vi "Verify Fiducial Positions.vi"(6 "Procedure Type":T1(ring)=enum."Gluing Verify Fiducials", 8 "error in":errorcluster, 9 "Path Fiducials":T8(array[cluster]), 10 "Module Fiducials":T6(array[cluster])) -> (0 "error out":errorcluster, 2 "All Good":bool)   [LabVIEW 2011]
uses:
  Shared Components/Utils/Type Definitions/Part Fiducials.ctl
  Shared Components/Utils/Type Definitions/Fiducial Image.ctl
  Shared Components/Vec3d Class/Vec3d Class.lvclass
  Shared Components/Utils/Type Definitions/Physical Image.ctl
  <vilib>/vision/Image Controls.llb/IMAQ Image.ctl
  Shared Components/Utils/Type Definitions/Fiducial with Source.ctl
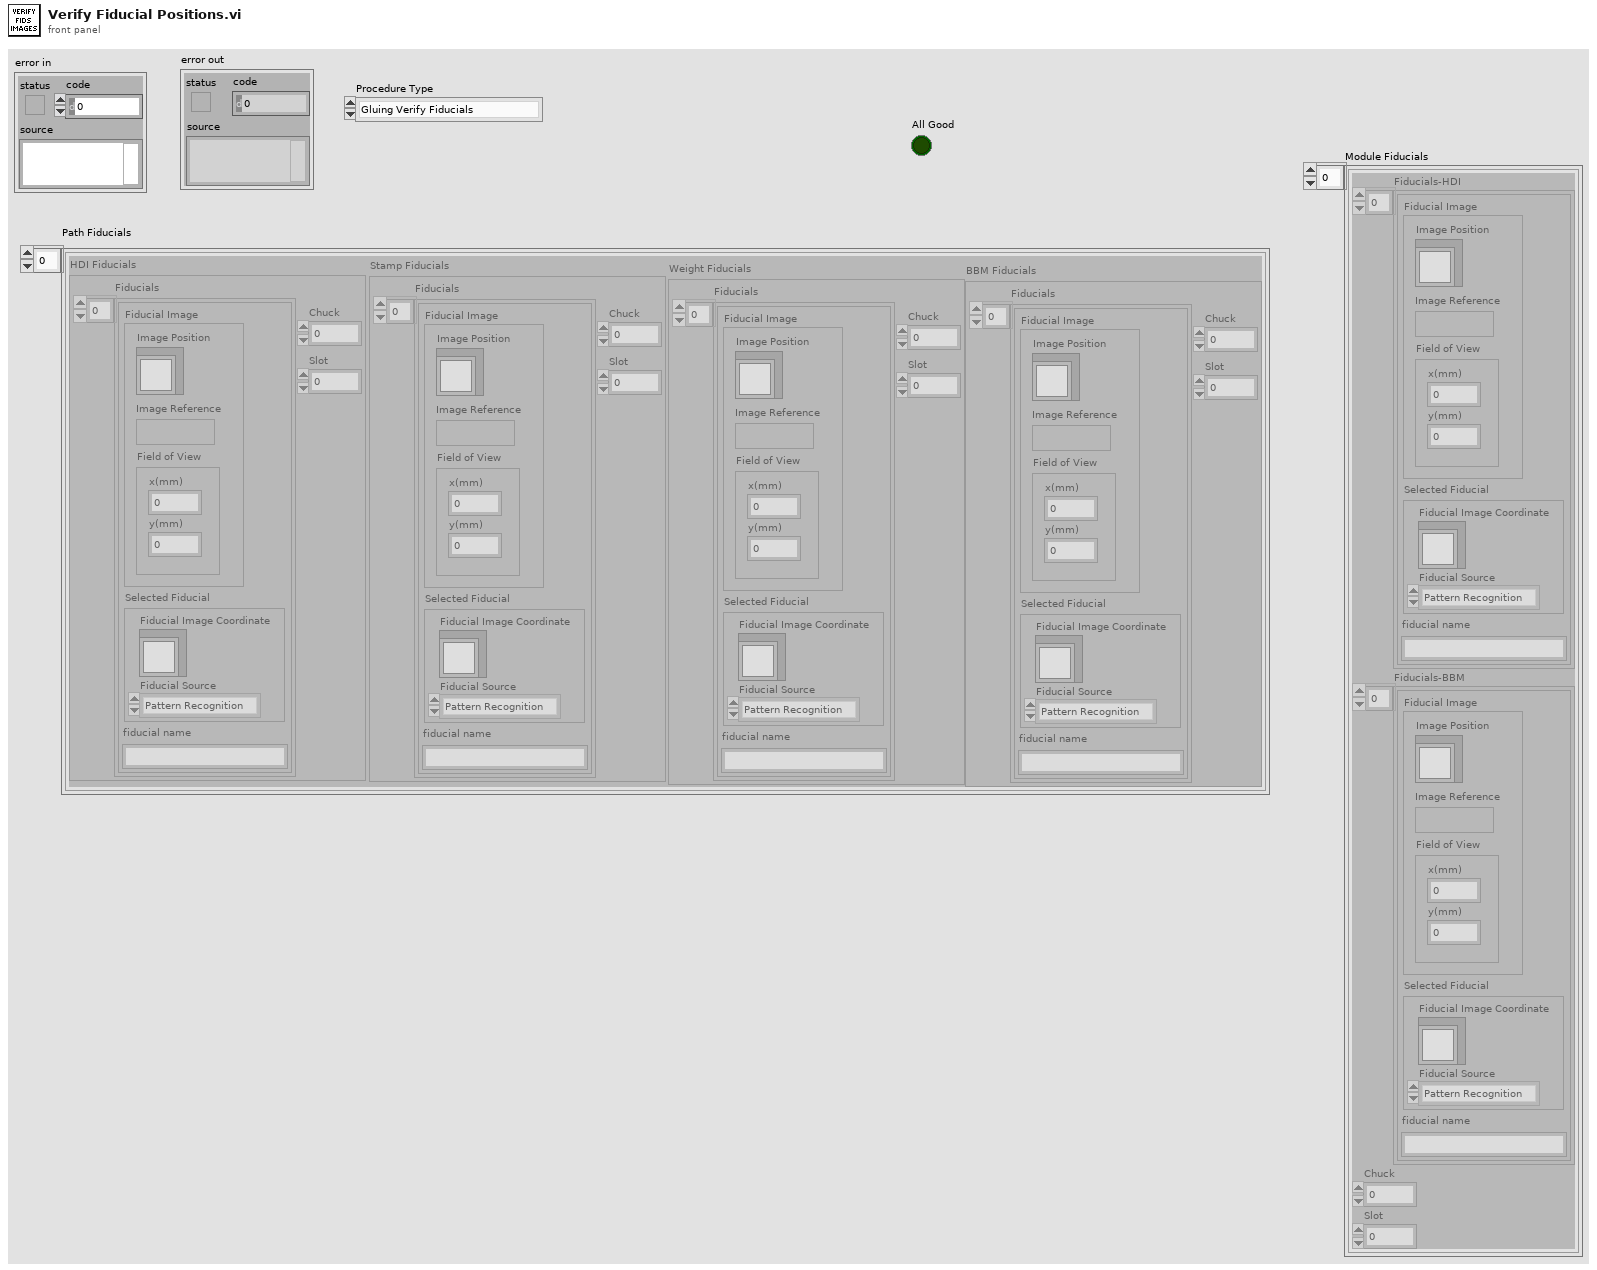
[diagram p1: front panel]
types:
  T1 = enum16{"Potting Verify Fiducials", "Gluing Verify Fiducials"}
  T2 = typedef "Fiducial Image.ctl" = cluster{"Fiducial Image":T3, "Selected Fiducial":T5, "fiducial name":string}
  T3 = typedef "Physical Image.ctl" = cluster{"Image Position":refnum<class "Vec3d Class.lvclass">, "Image Reference":T4, "Field of View":cluster{"x(mm)":dbl, "y(mm)":dbl}}
  T4 = typedef "IMAQ Image.ctl" = refnum<image>
  T5 = typedef "Fiducial with Source.ctl" = cluster{"Fiducial Image Coordinate":refnum<class "Vec3d Class.lvclass">, "Fiducial Source":enum16{"Pattern Recognition", "User", "Error", "Default"}}
  T6 = cluster{"Fiducials-HDI":T2[], "Fiducials-BBM":T2[], "Chuck":i32, "Slot":i32}[]
  T7 = typedef "Part Fiducials.ctl" = cluster{"Fiducials":T2[], "Chuck":i32, "Slot":i32}
  T8 = cluster{"HDI Fiducials":T7, "Stamp Fiducials":T7, "Weight Fiducials":T7, "BBM Fiducials":T7}[]
  T9 = enum16{"Pattern Recognition", "User", "Error", "Default"}
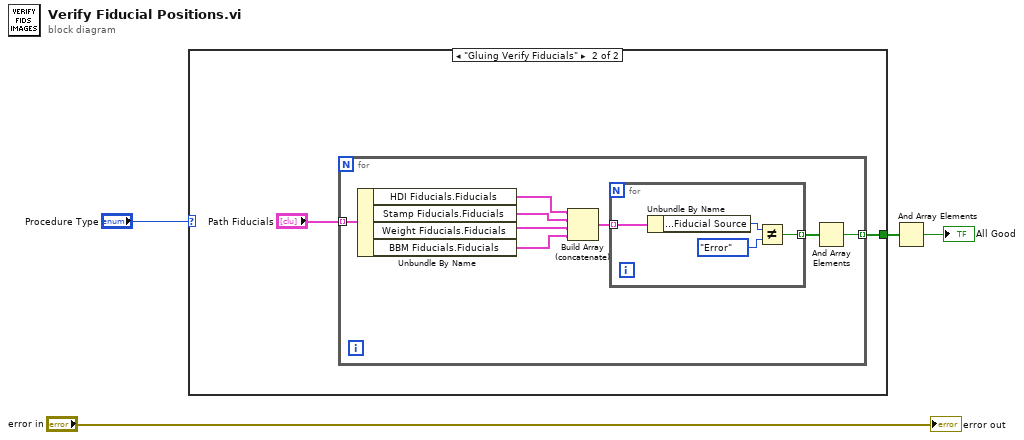
[diagram p0: block diagram]
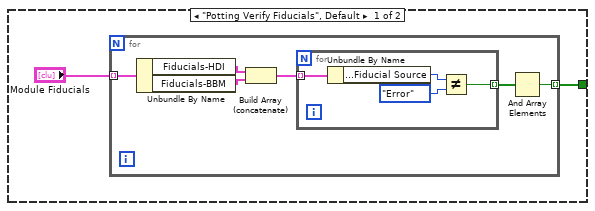
[diagram p2: hidden frame]
diagram:
  n1 = case shown="\"Gluing Verify Fiducials\"" "Procedure Type" {
    tunnel: [w5 w17] -> w3
    frame "Potting Verify Fiducials", Default {
      n2 = for {
        tunnel: "Module Fiducials" -> [w12] mode=indexing
        tunnel: [w7] -> w5 mode=indexing
        n3 = Unbundle By Name(w12) -> ("Fiducials-HDI"=w11:T2[], "Fiducials-BBM"=w10:T2[])
        n4 = Build Array (concatenate)(w11, w10) -> (w9:T2[])
        n5 = for {
          tunnel: w9 -> [w16] mode=indexing
          tunnel: [w14] -> w8 mode=indexing
          n6 = Unbundle By Name(w16) -> ("Selected Fiducial.Fiducial Source"=w15:T9)
          n7 = Not Equal?(x=w15, y=T9."Error") -> (x != y?=w14:bool)
        }
        n8 = And Array Elements(Boolean array=w8) -> (logical AND=w7:bool)
      }
    }
    frame "Gluing Verify Fiducials" {
      n9 = for {
        tunnel: "Path Fiducials" -> [w26] mode=indexing
        tunnel: [w19] -> w17 mode=indexing
        n10 = Unbundle By Name(w26) -> ("HDI Fiducials.Fiducials"=w25:T2[], "Stamp Fiducials.Fiducials"=w24:T2[], "Weight Fiducials.Fiducials"=w23:T2[], "BBM Fiducials.Fiducials"=w22:T2[])
        n11 = Build Array (concatenate)(w25, w24, w23, w22) -> (w21:T2[])
        n12 = for {
          tunnel: w21 -> [w30] mode=indexing
          tunnel: [w27] -> w20 mode=indexing
          n13 = Unbundle By Name(w30) -> ("Selected Fiducial.Fiducial Source"=w29:T9)
          n14 = Not Equal?(x=w29, y=T9."Error") -> (x != y?=w27:bool)
        }
        n15 = And Array Elements(Boolean array=w20) -> (logical AND=w19:bool)
      }
    }
  }
  n16 = And Array Elements(Boolean array=w3) -> (logical AND=→"All Good":bool)
  "error out" <- "error in"
